vi "Create(Configurable).vi"(5 "ConfigManager":refnum<class "ConfigManager.lvclass">, 7 "Shared Resource (F)":bool, 8 "error in (no error)":errorcluster, 10 "Subsystem Name (optional)":string, 11 "SMO":refnum<class "SMO.lvclass">) -> (0 "error out":errorcluster, 2 "SMO name":string, 3 "SMO out":refnum<class "SMO.lvclass">)   [LabVIEW 2013, in "SMO.lvclass"]
doc: "Constructor\n\n\n---------------------------------------------------------------\nJKI State Machine Objects™\nhttp://jki.net/state-machine-objects/\nCopyright (C) 2005-2015, JKI <info@jki.net>\nALL RIGHTS RESERVED"
uses:
  SMO.lvclass
  <vilib>/LabVIEW Open Source Project/Configuration Manager/Manager/ConfigManager.lvclass
panel:
  # "For instructions on how to use the JKI State Machine Objects, examples and video tutorials, visit:\nhttp://jki.net/state-machine-objects/\n\nJKI State Machine Objects™\nhttp://jki.net/state-machine-objects/\nCopyright (C) 2005-2015, JKI <info@jki.net>\nALL RIGHTS RESERVED"
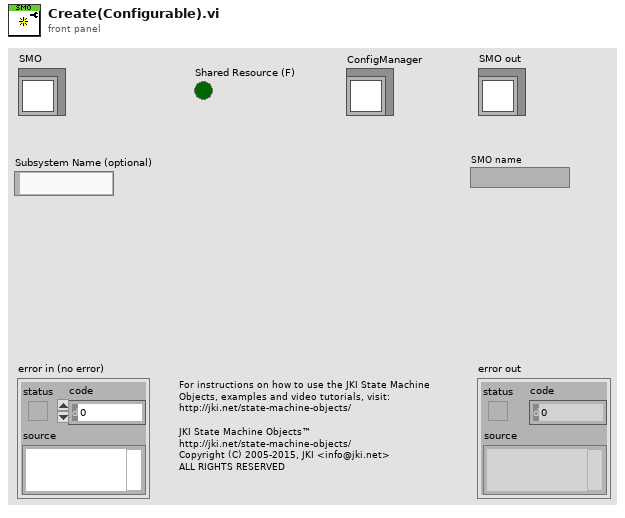
[diagram p1: front panel]
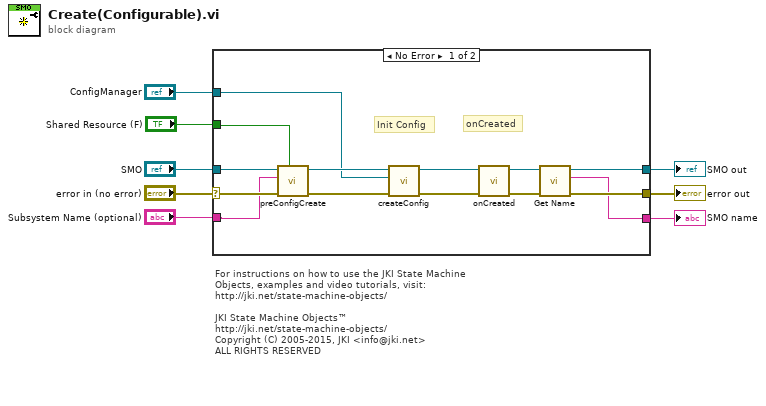
[diagram p0: block diagram]
diagram:
  # "For instructions on how to use the JKI State Machine Objects, examples and video tutorials, visit:\nhttp://jki.net/state-machine-objects/\n\nJKI State Machine Objects™\nhttp://jki.net/state-machine-objects/\nCopyright (C) 2005-2015, JKI <info@jki.net>\nALL RIGHTS RESERVED"
  n1 = case shown="No Error" "error in (no error)" {
    selector: "error in (no error)" -> [w16 w24]
    tunnel: [w19 w24] -> w2
    tunnel: [w21 w23] -> w3
    tunnel: "SMO" -> [w17 w23]
    tunnel: "Subsystem Name (optional)" -> [w15 _]
    tunnel: [w18 _] -> w1
    tunnel: "Shared Resource (F)" -> [w12 _]
    tunnel: "ConfigManager" -> [w9 _]
    frame No Error {
      # "Init Config"
      # "onCreated"
      n2 = call "preConfigCreate.vi"("Shared Resource (F)"=w12, "error in (no error)"=w16, "Subsystem Name (optional)"=w15, "SMO in"=w17) -> ("error out"=w14:errorcluster, "SMO out"=w13:refnum<class "SMO.lvclass">)  [unwired: 6 in]
      n3 = call "createConfig.vi"("error in (no error)"=w14, "SMOConfigManager"=w9, "SMO in"=w13) -> ("error out"=w10:errorcluster, "SMO out"=w11:refnum<class "SMO.lvclass">)  [unwired: 7 in]
      n4 = call-dynamic "onCreated.vi"("error in (no error)"=w10, "SMO"=w11) -> ("error out"=w20:errorcluster, "SMO out"=w22:refnum<class "SMO.lvclass">)  [unwired: 8 in]
      n5 = call "Get Name.vi"("error in (no error)"=w20, "SMO"=w22) -> ("error out"=w19:errorcluster, "Name"=w18:string, "SMO out"=w21:refnum<class "SMO.lvclass">)  [unwired: 5 in, 2 out]
    }
    frame Error {
    }
  }
  "error out" <- w2
  "SMO out" <- w3
  "SMO name" <- w1
